vi "周期测量_低频.vi"() -> ()   [LabVIEW 2013]
uses:
  <userlib>/ArtDAQ/_SubVI/ArtDAQ_CreateCIPeriodChan.vi
  <userlib>/ArtDAQ/_SubVI/ArtDAQ_Read Counter DBL 1Samp.vi
panel:
  out "数据":dbl
  in  "计数器":string="Dev1/ctr0"
  in  "最小值":dbl=1e-06 format="%0.6f"
  in  "MaxValue":dbl=10.0 caption="最大值" format="%0.6f"
  out "错误输出":errorcluster
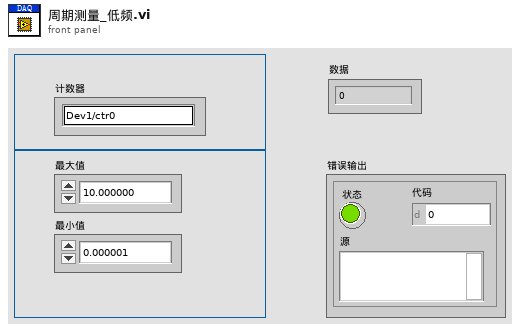
[diagram p1: front panel]
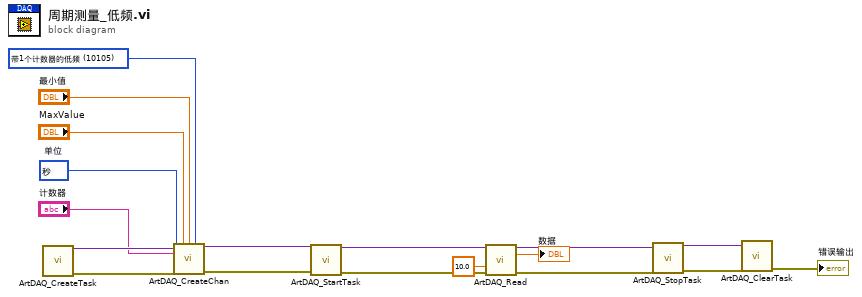
[diagram p0: block diagram]
diagram:
  w5 = 10105 items=["带1个计数器的低频"=10105, "带2个计数器的高频"=10157, "带2个计数器的大范围"=10205] ("测量方法")
  w6 = 10364 items=["秒"=10364, "时钟滴答"=10304, "来自自定义换算"=10065]  # 单位
  n1 = call <userlib>:"ArtDAQ_CreateTask.vi"() -> ("任务句柄"=w18:variant, "错误输出"=w17:errorcluster)  [unwired: 14 in]
  n2 = call-poly <userlib>:"ArtDAQ_CreateChan.vi"("任务句柄"=w18, "最大值"="MaxValue", "最小值"="最小值", "测量方法"=w5, "计数器"="计数器", "单位"=w6, "错误输入"=w17) -> ("任务句柄"=w4:variant, "错误输出"=w3:errorcluster)  [unwired: 7 in]
  n3 = call <userlib>:"ArtDAQ_StartTask.vi"("任务句柄"=w4, "错误输入"=w3) -> ("任务句柄"=w10:variant, "错误输出"=w9:errorcluster)  [unwired: 12 in]
  n4 = call-poly <userlib>:"ArtDAQ_Read.vi"("任务句柄"=w10, "超时s"=10.0 ("Timeout"), "错误输入"=w9) -> ("任务句柄"=w15:variant, "数据"=→"数据":dbl, "错误输出"=w13:errorcluster)  [unwired: 10 in]
  n5 = call <userlib>:"ArtDAQ_StopTask.vi"("任务句柄"=w15, "错误输入"=w13) -> ("任务句柄"=w14:variant, "错误输出"=w12:errorcluster)  [unwired: 12 in]
  n6 = call <userlib>:"ArtDAQ_ClearTask.vi"("任务句柄"=w14, "错误输入"=w12) -> ("错误输出"=→"错误输出":errorcluster)  [unwired: 13 in]
